vi "Init Bfr Rx - Data.vi"(7 "Data Access":refnum<class "Data Access Engine.lvclass">, 8 "error in (no error)":errorcluster, 11 "Parameters":variant) -> (0 "error out":errorcluster, 3 "Rx Loop Data":T1 {"Buffer Resources"."Data Buffer" format="%016x"; "Buffer Option Support"."Ping Pong Buffer"."Active Buffer Ref" format="%016x"; "Buffer Option Support"."Cached Buffer"."Cache Buffer" format="%016x"})   [LabVIEW 2019, in "UDP-Custom-Device Engine.lvlib"]
uses:
  UDP-Custom-Device Engine.lvlib
  <vilib>/NI/NIVS Inline Async API/_Data Access Engine/Data Access Engine/Data Access Engine.lvclass
  Types/Engine - Buffered Rx Loop Data.ctl
  Types/Engine - General Resources.ctl
  <vilib>/NI VeriStand/VeriStand Data/Typedefs/Typedefs.Data Types.ctl
  Shared/Types/Shared - Duplex Settings.ctl
  Shared/Types/Shared - Header Details.ctl
  Types/Engine - Buffer Resources.ctl
  Shared/Types/Shared - Pointer Encoding.ctl
  Types/Engine - Rx Runtime Resources.ctl
  Types/Engine - Execution Config.ctl
  Shared/Types/Shared - Thread Management.ctl
  Types/Engine - Rx New Data Options Support.ctl
  Shared/Types/Shared - New Data Options.ctl
  Types/Engine - Buffered Rx Buffer Option Support.ctl
  Shared/Types/Shared - Receive Buffer Options.ctl
  Types/Engine - Buffered Rx Circular Buffer.ctl
  Types/Engine - Buffered Rx Cached Buffer.ctl
  Types/Engine - Buffered Rx Ping Pong Buffer.ctl
  Types/Engine - Buffered Rx Active Buffer.ctl
  Types/Engine - Buffered Rx Channel Refs.ctl
  <vilib>/NI/NIVS Inline Async API/_Data Access Engine/Data Access Engine/Types/Write.DVR.ctl
  <vilib>/NI/NIVS Inline Async API/_Data Access Engine/Access Type Classes/Write/Write.lvclass
  <vilib>/NI/NIVS Inline Async API/_Data Access Engine/Data Access Engine/Types/Read.DVR.ctl
  <vilib>/NI/NIVS Inline Async API/_Data Access Engine/Access Type Classes/Read/Read.lvclass
  Types/Engine - Buffered Rx Ping Pong Channels.ctl
  Types/Engine - Debug Resources.ctl
  Shared/Types/Shared - Rx.PacketInfo.ctl
  Shared/Types/Shared - Channel Data Type.ctl
  Shared/Types/Shared - Buffered.PacketInfo.ctl
  Shared/Types/Shared - Transmit Buffer Options.ctl
  Init Bfr Rx - Create Option Channels.vi
  <vilib>/NI/NIVS Inline Async API/_Data Access Engine/Data Access Engine/Methods/Data.Processes.Lookup.vi
  <vilib>/NI/NIVS Inline Async API/_Data Access Engine/Data Access Engine/Methods/Write.Lookup.vi
  <vilib>/NI/NIVS Inline Async API/_Data Access Engine/Data Access Engine/Methods/Read.Lookup.vi
  Shared/UDP-Custom-Device Shared.lvlib
  <vilib>/NI VeriStand/VeriStand Data/VeriStand Data.lvlib
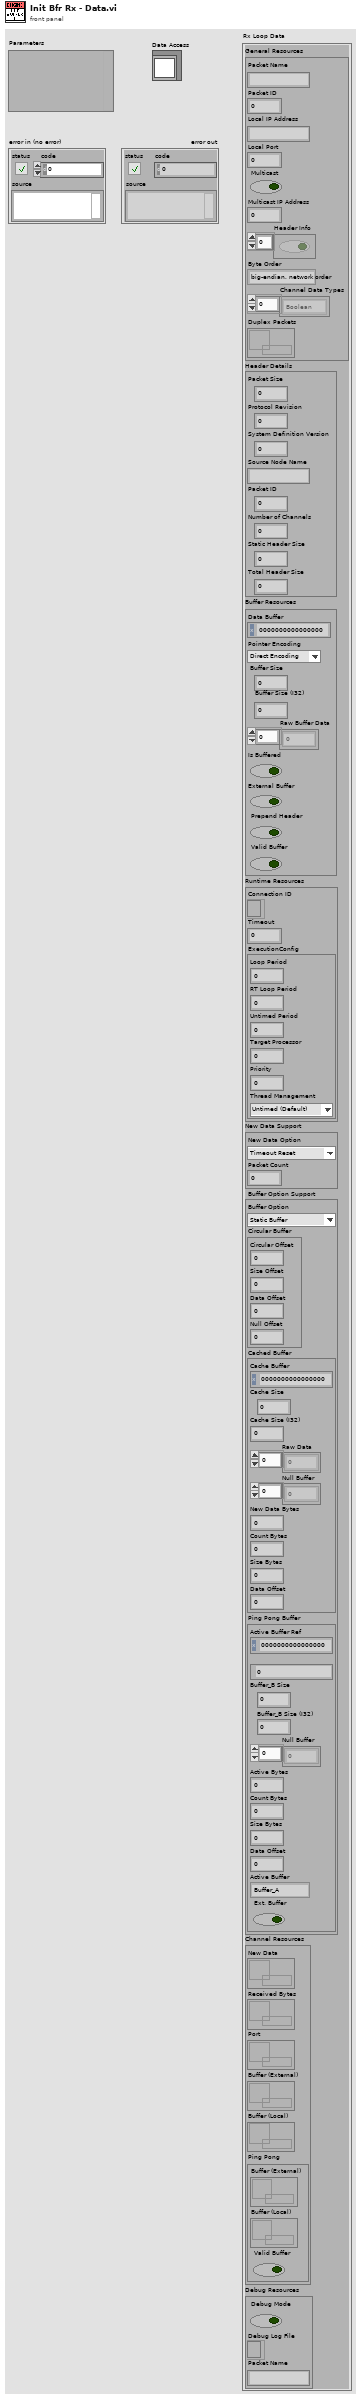
[diagram p1: front panel]
types:
  T1 = typedef "UDP-Custom-Device Engine.lvlib/Engine - Buffered Rx Loop Data.ctl" = cluster{"General Resources":T2, "Header Details":T4, "Buffer Resources":T5, "Runtime Resources":T7, "New Data Support":T10, "Buffer Option Support":T12, "Channel Resources":T18, "Debug Resources":T22}
  T2 = typedef "UDP-Custom-Device Engine.lvlib/Engine - General Resources.ctl" = cluster{"Packet Name":string, "Packet ID":i32, "Local IP Address":string, "Local Port":i32, "Multicast":bool, "Multicast IP Address":u32, "Header Info":bool[], "Byte Order":enum16{"big-endian, network order", "native, host order", "little-endian"}, "Channel Data Types":T3[], "Duplex Packets":refnum<data-value>}
  T3 = typedef "VeriStand Data.lvlib/Typedefs.Data Types.ctl" = enum16{"Boolean", "Single", "Double", "I8", "I16", "I32", "I64", "U8", "U16", "U32", "U64"}
  T4 = typedef "UDP-Custom-Device Shared.lvlib/Shared - Header Details.ctl" = cluster{"Packet Size":u16, "Protocol Revision":u8, "System Definition Version":u64, "Source Node Name":string, "Packet ID":u32, "Number of Channels":u32, "Static Header Size":u16, "Total Header Size":u16}
  T5 = typedef "UDP-Custom-Device Engine.lvlib/Engine - Buffer Resources.ctl" = cluster{"Data Buffer":u64, "Pointer Encoding":T6, "Buffer Size":u64, "Buffer Size (I32)":i32, "Raw Buffer Data":u8[], "Is Buffered":bool, "External Buffer":bool, "Prepend Header":bool, "Valid Buffer":bool}
  T6 = typedef "UDP-Custom-Device Shared.lvlib/Shared - Pointer Encoding.ctl" = enum16{"Direct Encoding", "Conversion Encoding"}
  T7 = typedef "UDP-Custom-Device Engine.lvlib/Engine - Rx Runtime Resources.ctl" = cluster{"Connection ID":refnum<k16>, "Timeout":i32, "ExecutionConfig":T8}
  T8 = typedef "UDP-Custom-Device Engine.lvlib/Engine - Execution Config.ctl" = cluster{"Loop Period":i64, "RT Loop Period":i64, "Untimed Period":u32, "Target Processor":i32, "Priority":i32, "Thread Management":T9}
  T9 = typedef "UDP-Custom-Device Shared.lvlib/Shared - Thread Management.ctl" = enum16{"Untimed (Default)", "Timed (High Priority)"}
  T10 = typedef "UDP-Custom-Device Engine.lvlib/Engine - Rx New Data Options Support.ctl" = cluster{"New Data Option":T11, "Packet Count":dbl}
  T11 = typedef "UDP-Custom-Device Shared.lvlib/Shared - New Data Options.ctl" = enum16{"Timeout Reset", "Counter"}
  T12 = typedef "UDP-Custom-Device Engine.lvlib/Engine - Buffered Rx Buffer Option Support.ctl" = cluster{"Buffer Option":T13, "Circular Buffer":T14, "Cached Buffer":T15, "Ping Pong Buffer":T16}
  T13 = typedef "UDP-Custom-Device Shared.lvlib/Shared - Receive Buffer Options.ctl" = enum16{"Static Buffer", "Circular Buffer", "Circular Buffer + Size", "Internal Cache", "Internal Cache + Size", "Ping Pong", "Ping Pong + Size"}
  T14 = typedef "UDP-Custom-Device Engine.lvlib/Engine - Buffered Rx Circular Buffer.ctl" = cluster{"Circular Offset":u64, "Size Offset":u64, "Data Offset":u64, "Null Offset":u64}
  T15 = typedef "UDP-Custom-Device Engine.lvlib/Engine - Buffered Rx Cached Buffer.ctl" = cluster{"Cache Buffer":u64, "Cache Size":u64, "Cache Size (I32)":i32, "Raw Data":u8[], "Null Buffer":u8[], "New Data Bytes":u64, "Count Bytes":u64, "Size Bytes":u64, "Data Offset":u64}
  T16 = typedef "UDP-Custom-Device Engine.lvlib/Engine - Buffered Rx Ping Pong Buffer.ctl" = cluster{"Active Buffer Ref":u64, "Buffer_B":u64, "Buffer_B Size":u64, "Buffer_B Size (I32)":i32, "Null Buffer":u8[], "Active Bytes":u64, "Count Bytes":u64, "Size Bytes":u64, "Data Offset":u64, "Active Buffer":T17, "Ext. Buffer":bool}
  T17 = typedef "UDP-Custom-Device Engine.lvlib/Engine - Buffered Rx Active Buffer.ctl" = enum16{"Buffer_A", "Buffer_B"}
  T18 = typedef "UDP-Custom-Device Engine.lvlib/Engine - Buffered Rx Channel Refs.ctl" = cluster{"New Data":T19, "Received Bytes":T19, "Port":T19, "Buffer (External)":T20, "Buffer (Local)":T19, "Ping Pong":T21}
  T19 = typedef "Data Access Engine.lvlib/Data Access Engine.lvclass/Write.DVR.ctl" = refnum<data-value>
  T20 = typedef "Data Access Engine.lvlib/Data Access Engine.lvclass/Read.DVR.ctl" = refnum<data-value>
  T21 = typedef "UDP-Custom-Device Engine.lvlib/Engine - Buffered Rx Ping Pong Channels.ctl" = cluster{"Buffer (External)":T20, "Buffer (Local)":T19, "Valid Buffer":bool}
  T22 = typedef "UDP-Custom-Device Engine.lvlib/Engine - Debug Resources.ctl" = cluster{"Debug Mode":bool, "Debug Log File":refnum<file>, "Packet Name":string}
  T23 = typedef "UDP-Custom-Device Shared.lvlib/Shared - Rx.PacketInfo.ctl" = cluster{"Packet Name":string, "Packet ID":i32, "Timeout":i32, "Rx IP Address":string, "Rx Port":u16, "Endianness":u16, "Multicast":bool, "Multicast IP Address":string, "Diagnostics En?":bool, "Debug Mode":bool, "Header Info":bool[], "Channel Data Types":T24[], "Buffered Packet Info":T25, "Duplex Packets":refnum<data-value>, "New Data Option":T11, "targetPriority":i16, "targetProcessor":i8, "Thread Management":T9}
  T24 = typedef "UDP-Custom-Device Shared.lvlib/Shared - Channel Data Type.ctl" = enum16{"Boolean", "Single", "Double", "I8", "I16", "I32", "I64", "U8", "U16", "U32", "U64"}
  T25 = typedef "UDP-Custom-Device Shared.lvlib/Shared - Buffered.PacketInfo.ctl" = cluster{"Buffer Size":i32, "External Buffer":bool, "Prepend Header":bool, "Is Buffered":bool, "Pointer Encoding":T6, "Rx Buffer Option":T13, "Tx Buffer Option":T26}
  T26 = typedef "UDP-Custom-Device Shared.lvlib/Shared - Transmit Buffer Options.ctl" = enum16{"Static Buffer", "FIFO Buffer", "FIFO Buffer + Port"}
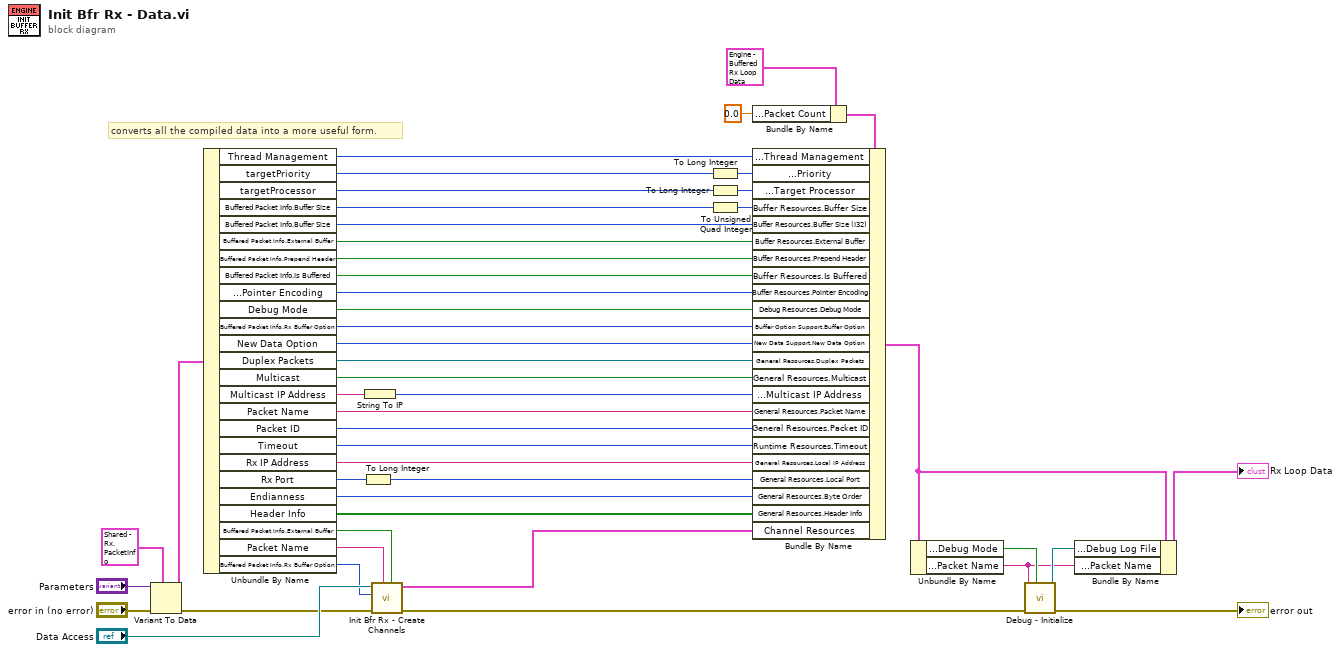
[diagram p0: block diagram]
diagram:
  # "converts all the compiled data into a more useful form."
  n1 = Variant To Data(error in="error in (no error)", type=T23 {"Packet Name"="", "Packet ID"=0, "Timeout"=0, "Rx IP Address"="", "Rx Port"=0, "Endianness"=0, "Multicast"=FALSE, "Multicast IP Address"="", "Diagnostics En?"=FALSE, "Debug Mode"=FALSE, "Header Info"=[], "Channel Data Types"=[], "Buffered Packet Info"={"Buffer Size"=0, "External Buffer"=FALSE, "Prepend Header"=FALSE, "Is Buffered"=FALSE, "Pointer Encoding"=enum."Direct Encoding", "Rx Buffer Option"=enum."Static Buffer", "Tx Buffer Option"=enum."Static Buffer"}, "Duplex Packets"=refnum, "New Data Option"=enum."Timeout Reset", "targetPriority"=1, "targetProcessor"=0, "Thread Management"=enum."Untimed (Default)"} ("Rx Packet Info"), Variant="Parameters") -> (data=w44:T23, error out=w7:errorcluster)
  n2 = Unbundle By Name(w44) -> ("Thread Management"=w11:T9, "targetPriority"=w15:i16, "targetProcessor"=w14:i8, "Buffered Packet Info.Buffer Size"=w16:i32, "Buffered Packet Info.Buffer Size"=w2:i32, "Buffered Packet Info.External Buffer"=w20:bool, "Buffered Packet Info.Prepend Header"=w21:bool, "Buffered Packet Info.Is Buffered"=w22:bool, "Buffered Packet Info.Pointer Encoding"=w23:T6, "Debug Mode"=w29:bool, "Buffered Packet Info.Rx Buffer Option"=w30:T13, "New Data Option"=w31:T11, "Duplex Packets"=w32:refnum<data-value>, "Multicast"=w35:bool, "Multicast IP Address"=w34:string, "Packet Name"=w43:string, "Packet ID"=w42:i32, "Timeout"=w36:i32, "Rx IP Address"=w41:string, "Rx Port"=w40:u16, "Endianness"=w38:u16, "Header Info"=w37:bool[], "Buffered Packet Info.External Buffer"=w5:bool, "Packet Name"=w6:string, "Buffered Packet Info.Rx Buffer Option"=w1:T13)
  n3 = To Long Integer(number=w40) -> (32bit integer=w39:i32)
  n4 = String To IP(1:w34) -> (0:w33:u32)
  n5 = call "Init Bfr Rx - Create Channels.vi"("External Buffer"=w5, "Packet Name"=w6, "error in (no error)"=w7, "Rx Buffer Option"=w1, "Data Access"="Data Access") -> ("error out"=w3:errorcluster, "Buffered Receive Channels"=w4:T18)  [unwired: 5 in]
  n6 = To Long Integer(number=w15) -> (32bit integer=w12:i32)
  n7 = To Long Integer(number=w14) -> (32bit integer=w13:i32)
  n8 = To Unsigned Quad Integer(1:w16) -> (0:w10:u64)
  n9 = Bundle By Name(cluster=T1 {"General Resources"={"Packet Name"="", "Packet ID"=0, "Local IP Address"="", "Local Port"=0, "Multicast"=FALSE, "Multicast IP Address"=0, "Header Info"=[], "Byte Order"=enum."big-endian, network order", "Channel Data Types"=[], "Duplex Packets"=refnum}, "Header Details"={"Packet Size"=0, "Protocol Revision"=0, "System Definition Version"=0, "Source Node Name"="", "Packet ID"=0, "Number of Channels"=0, "Static Header Size"=0, "Total Header Size"=0}, "Buffer Resources"={"Data Buffer"=0, "Pointer Encoding"=enum."Direct Encoding", "Buffer Size"=0, "Buffer Size (I32)"=0, "Raw Buffer Data"=[], "Is Buffered"=FALSE, "External Buffer"=FALSE, "Prepend Header"=FALSE, "Valid Buffer"=FALSE}, "Runtime Resources"={"Connection ID"=refnum, "Timeout"=0, "ExecutionConfig"={"Loop Period"=0, "RT Loop Period"=0, "Untimed Period"=0, "Target Processor"=0, "Priority"=0, "Thread Management"=enum."Untimed (Default)"}}, "New Data Support"={"New Data Option"=enum."Timeout Reset", "Packet Count"=0.0}, "Buffer Option Support"={"Buffer Option"=enum."Static Buffer", "Circular Buffer"={"Circular Offset"=0, "Size Offset"=0, "Data Offset"=0, "Null Offset"=0}, "Cached Buffer"={"Cache Buffer"=0, "Cache Size"=0, "Cache Size (I32)"=0, "Raw Data"=[], "Null Buffer"=[], "New Data Bytes"=0, "Count Bytes"=0, "Size Bytes"=0, "Data Offset"=0}, "Ping Pong Buffer"={"Active Buffer Ref"=0, "Buffer_B"=0, "Buffer_B Size"=0, "Buffer_B Size (I32)"=0, "Null Buffer"=[], "Active Bytes"=0, "Count Bytes"=0, "Size Bytes"=0, "Data Offset"=0, "Active Buffer"=enum."Buffer_A", "Ext. Buffer"=FALSE}}, "Channel Resources"={"New Data"=refnum, "Received Bytes"=refnum, "Port"=refnum, "Buffer (External)"=refnum, "Buffer (Local)"=refnum, "Ping Pong"={"Buffer (External)"=refnum, "Buffer (Local)"=refnum, "Valid Buffer"=FALSE}}, "Debug Resources"={"Debug Mode"=FALSE, "Debug Log File"=refnum, "Packet Name"=""}} ("Rx Loop Data"), "New Data Support.Packet Count"=0.0) -> (w18:T1)
  n10 = Bundle By Name(cluster=w18, "Runtime Resources.ExecutionConfig.Thread Management"=w11, "Runtime Resources.ExecutionConfig.Priority"=w12, "Runtime Resources.ExecutionConfig.Target Processor"=w13, "Buffer Resources.Buffer Size"=w10, "Buffer Resources.Buffer Size (I32)"=w2, "Buffer Resources.External Buffer"=w20, "Buffer Resources.Prepend Header"=w21, "Buffer Resources.Is Buffered"=w22, "Buffer Resources.Pointer Encoding"=w23, "Debug Resources.Debug Mode"=w29, "Buffer Option Support.Buffer Option"=w30, "New Data Support.New Data Option"=w31, "General Resources.Duplex Packets"=w32, "General Resources.Multicast"=w35, "General Resources.Multicast IP Address"=w33, "General Resources.Packet Name"=w43, "General Resources.Packet ID"=w42, "Runtime Resources.Timeout"=w36, "General Resources.Local IP Address"=w41, "General Resources.Local Port"=w39, "General Resources.Byte Order"=w38, "General Resources.Header Info"=w37, "Channel Resources"=w4) -> (w9:T1)
  n11 = Unbundle By Name(w9) -> ("Debug Resources.Debug Mode"=w28:bool, "General Resources.Packet Name"=w24:string)
  n12 = call "Debug - Initialize.vi"("Debug Mode"=w28, "error in (no error)"=w3, "Packet Name"=w24) -> ("error out"=→"error out":errorcluster, "Debug Log File"=w27:refnum<file>)  [unwired: 7 in]
  n13 = Bundle By Name(cluster=w9, "Debug Resources.Debug Log File"=w27, "Debug Resources.Packet Name"=w24) -> (→"Rx Loop Data":T1)
